vi "SetupCLStim_2Analog.vi"(0 "event port":u16=5557, 1 "Sham stim event channel":u16=3 min=1 max=8, 2 "Real stim channel":tag="pciDAQ/ao0", 3 "Sham stim channel":tag="pciDAQ/ao2", 4 "OEP sample clock in":tag="/pciDAQ/PFI0", 5 "Onboard counter":tag="pciDAQ/ctr0") -> (9 "ZMQ error out":errorcluster, 10 "context out":refnum<class "zmq_context.lvclass">, 11 "socket out":refnum<class "zmq_socket.lvclass">, 13 "clock offset":i64, 14 "Real stim task":refnum<k21>, 15 "Sham stim task":refnum<k21>, 16 "Waveform Graph":waveform(dbl)(graph), 18 "Ctr task":refnum<k21>, 19 "DAQ error out":errorcluster)   [LabVIEW 2017]
uses:
  <vilib>/addons/zeromq/zmq_socket.lvclass
  <vilib>/addons/zeromq/zmq_context.lvclass
  <vilib>/DAQmx/write.llb/DAQmx Write (Analog Wfm 1Chan NSamp).vi
  <vilib>/DAQmx/read.llb/DAQmx Read (Counter U32 1Chan 1Samp).vi
  <vilib>/addons/zeromq/zmq_recv_multi.vi
  <vilib>/DAQmx/miscellaneous.llb/DAQmx Fill In Error Info.vi
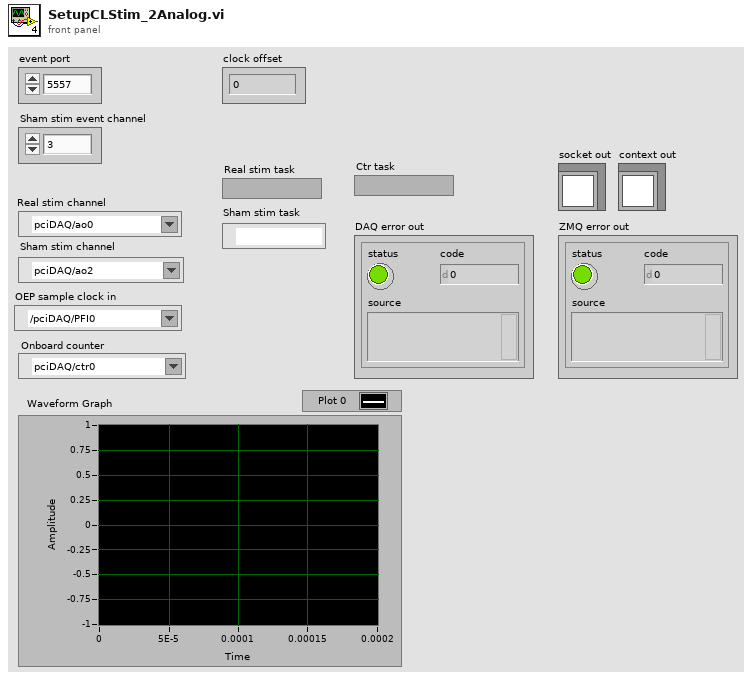
[diagram p1: front panel]
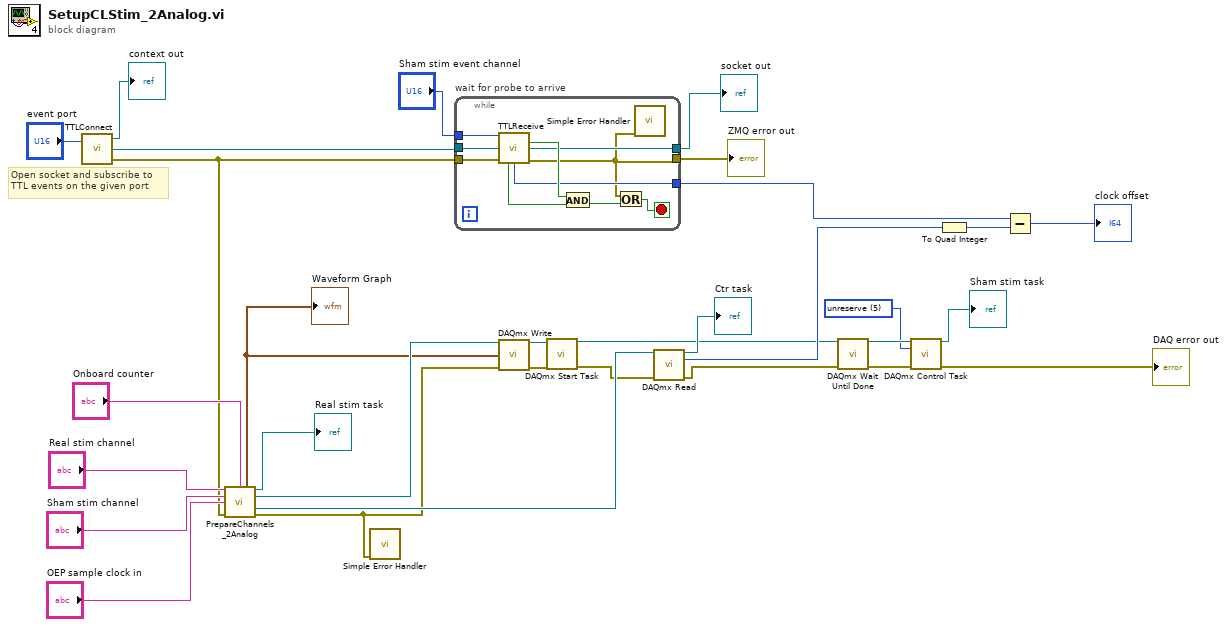
[diagram p0: block diagram]
diagram:
  w16 = 5 items=["verify"=2, "reserve"=4, "commit"=3, "unreserve"=5, "abort"=6] ("action")
  # "Open socket and subscribe to\nTTL events on the given port"
  n1 = call "TTLConnect.vi"("port"="event port") -> ("context out"=→"context out":refnum<class "zmq_context.lvclass">, "socket out"=w26:refnum<class "zmq_socket.lvclass">, "error out"=w5:errorcluster)  [unwired: 1 in]
  n2 = call "PrepareChannels_2Analog.vi"("Real stim channel"="Real stim channel", "Onboard counter"="Onboard counter", "Sham stim channel"="Sham stim channel", "OEP sample clock in"="OEP sample clock in", "error in"=w5) -> ("Waveform Graph"=w1:waveform(dbl), "Real stim task"=→"Real stim task":refnum<k21>, "Sham stim task"=w15:refnum<k21>, "ctr task out"=w14:refnum<k21>, "Error out"=w10:errorcluster)  [unwired: 6 in]
  "Waveform Graph" <- w1
  n3 = call <vilib>:"Simple Error Handler.vi"("error in (no error)"=w10) -> ()  [unwired: 4 in, 5 out]
  n4 = while "wait for probe to arrive" {
    tunnel: w26 -> [w41]
    tunnel: "Sham stim event channel" -> [w40]
    tunnel: [w37] -> w28
    tunnel: [w32] -> w23
    tunnel: [w36] -> w30
    tunnel: w5 -> [w35]
    stop <- w34 stop-if-true
    n5 = call "TTLReceive.vi"("channel"=w40, "socket in"=w41, "error in"=w35) -> ("new TTL"=w39:bool, "socket out"=w36:refnum<class "zmq_socket.lvclass">, "event on"=w38:bool, "timestamp"=w37:i64, "error out"=w32:errorcluster)  [unwired: 7 in, 1 out]
    n6 = And(x=w39, y=w38) -> (x .and. y?=w33:bool)
    n7 = Or(x=w32, y=w33) -> (x .or. y?=w34:bool)
    n8 = call <vilib>:"Simple Error Handler.vi"("error in (no error)"=w32) -> ()  [unwired: 4 in, 5 out]
  }
  "ZMQ error out" <- w23
  "socket out" <- w30
  n9 = call-poly <vilib>:"DAQmx Write.vi"("task/channels in"=w15, "data"=w1, "error in"=w10) -> ("task out"=w9:refnum<k21>, "error out"=w8:errorcluster)  [unwired: 10 in, 1 out]
  n10 = call <vilib>:"DAQmx Start Task.vi"("task/channels in"=w9, "error in"=w8) -> ("task out"=w6:refnum<k21>, "error out"=w11:errorcluster)  [unwired: 12 in]
  n11 = call-poly <vilib>:"DAQmx Read.vi"("task/channels in"=w14, "error in"=w11) -> ("task out"=→"Ctr task":refnum<k21>, "data"=w12:u32, "error out"=w7:errorcluster)  [unwired: 11 in]
  n12 = call <vilib>:"DAQmx Wait Until Done.vi"("task/channels in"=w6, "error in"=w7) -> ("task out"=w18:refnum<k21>, "error out"=w17:errorcluster)  [unwired: 12 in]
  n13 = call <vilib>:"DAQmx Control Task.vi"("task/channels in"=w18, "action"=w16, "error in"=w17) -> ("task out"=→"Sham stim task":refnum<k21>, "error out"=→"DAQ error out":errorcluster)  [unwired: 11 in]
  n14 = To Quad Integer(1:w12) -> (0:w31:i64)
  n15 = Subtract(x=w28, y=w31) -> (x-y=→"clock offset":i64)
